vi "Read States.vi"(8 "error in (no error)":errorcluster, 11 "ShootTactic in":refnum<class "ShootTactic.lvclass">) -> (0 "error out":errorcluster, 2 "States":T1=enum."KickToGoal", 3 "ShootTactic out":refnum<class "ShootTactic.lvclass">)   [LabVIEW 2018, in "ShootTactic.lvclass"]
uses:
  ShootTactic.lvclass
  States.ctl
  ShootTactic.lvclass/ShootTactic.ctl
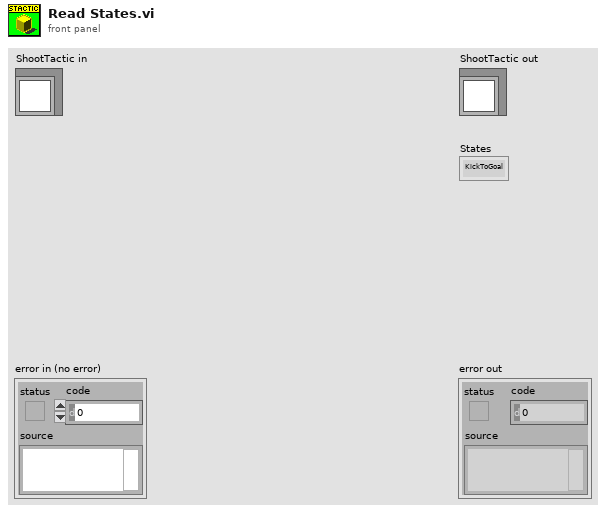
[diagram p1: front panel]
types:
  T1 = typedef "ShootTactic.lvclass/States.ctl" = enum16{"Exit", "KickToGoal", "StealBall"}
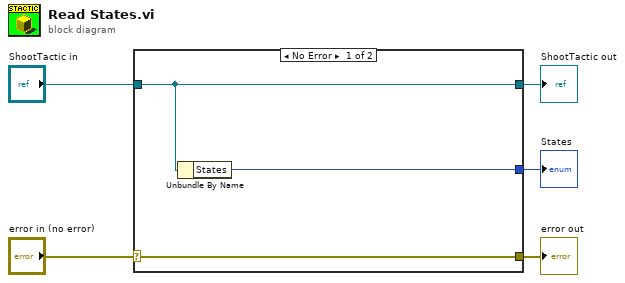
[diagram p0: block diagram]
diagram:
  n1 = case shown="No Error" "error in (no error)" {
    selector: "error in (no error)" -> [w8 w9]
    tunnel: [w8 w9] -> w4
    tunnel: [w7 w10] -> w2
    tunnel: "ShootTactic in" -> [w7 w10]
    tunnel: [w6 _] -> w1
    frame No Error {
      n2 = Unbundle By Name(w7) -> ("States"=w6:T1)
    }
    frame Error {
    }
  }
  "error out" <- w4
  "ShootTactic out" <- w2
  "States" <- w1
